vi "Dashboard Main.vi"() -> ()   [LabVIEW 2013]
uses:
  <vilib>/event_ctls.llb/eventvkey.ctl
  <vilib>/Rock Robotics/WPI/Dashboard/WPI_DashboardLogging Global.vi
  <vilib>/Utility/config.llb/Write Key (String).vi
  <vilib>/Utility/config.llb/Write Key (I32).vi
  <vilib>/Utility/config.llb/NI_LVConfig.lvlib
panel:
  out "JS2 Z 2":dbl(slide) scale=-1.0..1.0 scale format="%#_2e"
  out "Joystick 4":cluster{"X":dbl, "Y":dbl}[](graph)
  out "JS1 Z 2":dbl(slide) scale=-1.0..1.0 scale format="%#_2e"
  out "Joystick 3":cluster{"X":dbl, "Y":dbl}[](graph)
  out "code":string
  out "Image Message":string="Timeout in Camera Communications"
  in  "Rec Mode":enum32{"Stop", "Record", "Playback"}(radio)
  in  "Dashboard Tab":T1(tab)
  in  "Camera Settings":T2={"Frame Rate"=30, "Compression"=30, "Size"=1} {"Frame Rate" scale=1.0..30.0; "Size" items=["640x480", "320x240", "160x120"]}
  out "MotorSliders R":cluster{"MotorSlide1":dbl, "MotorSlide2":dbl} {"MotorSlide2" scale=-1.0..1.0 scale format="%#_2e"; "MotorSlide1" scale=-1.0..1.0 scale format="%#_2e"}
  out "MotorChart R":cluster{"Numeric":dbl, "Numeric":dbl}(graph)
  out "MotorSliders L":T3 {"MotorSlide4 2" scale=0.0..14.0 scale format="%#_2e"; "MotorSlide2" scale=-1.0..1.0 scale format="%#_2e"; "MotorSlide1" scale=-1.0..1.0 scale format="%#_2e"}
  out "MotorChart L":T4(graph)
  out "JS1 Z":dbl(slide) scale=-1.0..1.0 scale format="%#_2e"
  out "Joystick 1":cluster{"X":dbl, "Y":dbl}[](graph)
  out "JS Buttons 1":T5
  out "JS2 Z":dbl(slide) scale=-1.0..1.0 scale format="%#_2e"
  out "Joystick 2":cluster{"X":dbl, "Y":dbl}[](graph)
  out "JS Buttons 2":T5
  out "Mode":T6(ring)=enum."Auto Disabled"
  out "Camera IP":string
  in  "DB Camera Config":bool
  out "fps":dbl format="%#.1g"
  out "Mbps":dbl format="%#.1g"
  out "Mbps 2":bool
  out "LED 1":bool
  in  "loadCode":bool
  in  "pick auto":string
  out "Timer":dbl
  out "Mode 2":string
  out "left Encoder":dbl
  out "right Encoder":dbl
  out "Waveform Chart":T7(graph)
  out "Plot 0 Ind":dbl
  out "Plot 1 Ind":dbl
  out "Polt 2 Ind":dbl
  in  "Checkbox 2":bool
  in  "Checkbox 1":bool
  in  "Test Slider":dbl(slide) scale=0.0..100.0 scale format="%#_3g"
  in  "On/Off":bool caption="Solenoid"
  in  "Test Name":u16(ring) items=["Select the test to run...", "Example Test", "-------------------------------", "List of tests is built in robot code.", "Replace with your own automated tests."]
  in  "Test Tree":string(tree)
  in  "Motor":cluster{"Value":dbl, "Enable":bool} {"Value" scale=-1.0..1.0 scale format="%#_3g"}
  out "Progress":T8 {"Test Progress" scale=0.0..100.0}
  in  "Rev/Fwd":cluster{"Forward":bool, "Reverse":bool}
  in  "Test Ring":u16(ring) items=["Auto", "Fixed indoor", "Fixed outdoor 1", "Fixed outdoor 2", "Fixed fluorescent 1", "Fixed fluorescent 2", "Hold current"]
  in  "Listbox":i32(listbox)
  out "Tree":string(tree)
  out "Camera Image":T9(plugin-control)
  in  "Enable":bool
  # "Left"
  # "Front"
  # "Right"
  # "Battery"
  # "This tab is a great place for autonomous settings and validation.\nCustomize by placing controls and indicators here and name to\nmatch Dashboard Variables on robot."
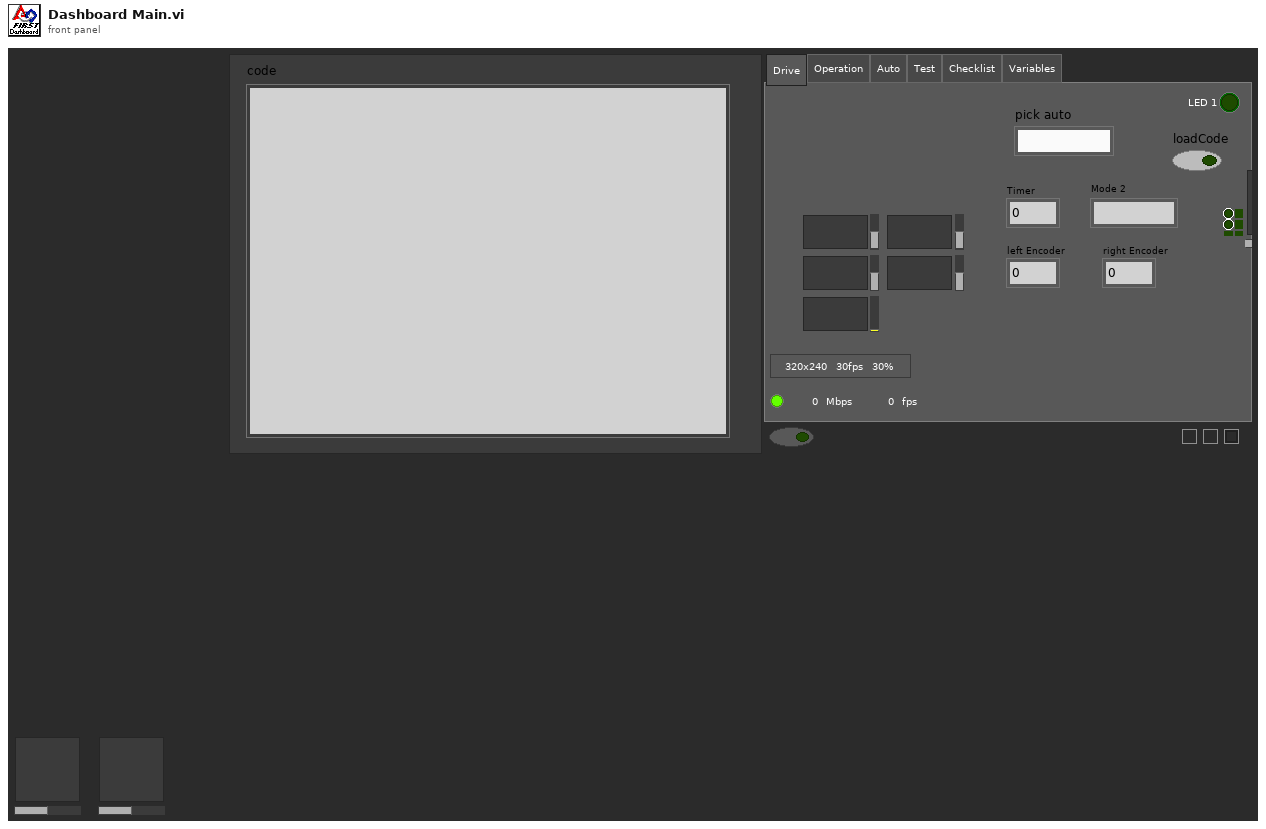
[diagram p1: front panel]
types:
  T1 = enum32{"Drive", "Operation", "Auto", "Test", "Checklist", "Variables"}
  T2 = cluster{"Frame Rate":i32, "Compression":i32, "Size":u16}
  T3 = cluster{"MotorSlide1":dbl, "MotorSlide2":dbl, "MotorSlide4 2":dbl}
  T4 = cluster{"Numeric":dbl, "Numeric":dbl, "Battery":sgl}
  T5 = cluster{bool, bool, bool, bool, bool, bool, bool, bool, bool, bool, bool, bool}
  T6 = enum8{"Tele-Op Disabled", "Tele-Op Enabled", "Auto Disabled", "Auto Enabled", "Test Disabled", "Test Enabled", ""}
  T7 = cluster{"Numeric":dbl, "Numeric":dbl, "Numeric":dbl}
  T8 = cluster{"Test Progress":u8, "Test Progress Text":string}
  T9 = typedef "IMAQ Image.ctl" = refnum<image>
  T10 = typedef "Image Type" = u32
  T11 = cluster{"Digital Inputs":bool[], "Digital Outputs":bool[]}
  T12 = cluster{"Competition mode":bool, "Robot Link":bool, "Autonomous":bool, "Enabled":bool, "E-Stop":bool, "Simulated":bool, "TestMode":bool, "Docked Window":bool}
  T13 = cluster{"Boolean":bool, "Boolean":bool, "Boolean":bool, "Boolean":bool, "Boolean":bool, "Boolean":bool, "Boolean":bool, "Boolean":bool, "Boolean":bool, "Boolean":bool, "Boolean":bool, "Boolean":bool}
  T14 = typedef "NI_LVConfig.lvlib/Config Data RefNum.ctl" = refnum<k1>
  T15 = typedef "eventvkey.ctl" = enum16{"ASCII", "Enter", "Return", "Shift", "Ctrl", "Alt", "Cmd", "Opt", "Caps", "NumLock", "Clear", "Break", "Up", "Down", "Left", "Right", "Insert", "Delete", "Home", "End", "PageUp", "PageDown", "Escape", "Help", "Pause", "ScrollLock", "F1", "F2", "F3", "F4", "F5", "F6", "F7", "F8", "F9", "F10", "F11", "F12", "F13", "F14", "F15", "F16", "F17", "F18", "F19", "F20", "F21", "F22", "F23", "F24", "Play", "VolumeUp", "VolumeDown", "Mute", "Two Byte Char"}
  T16 = cluster{"Image Size":bool, "Image Type":bool, "Pixel Value":bool, "ROI Information":bool, "Zoom Factor":bool}
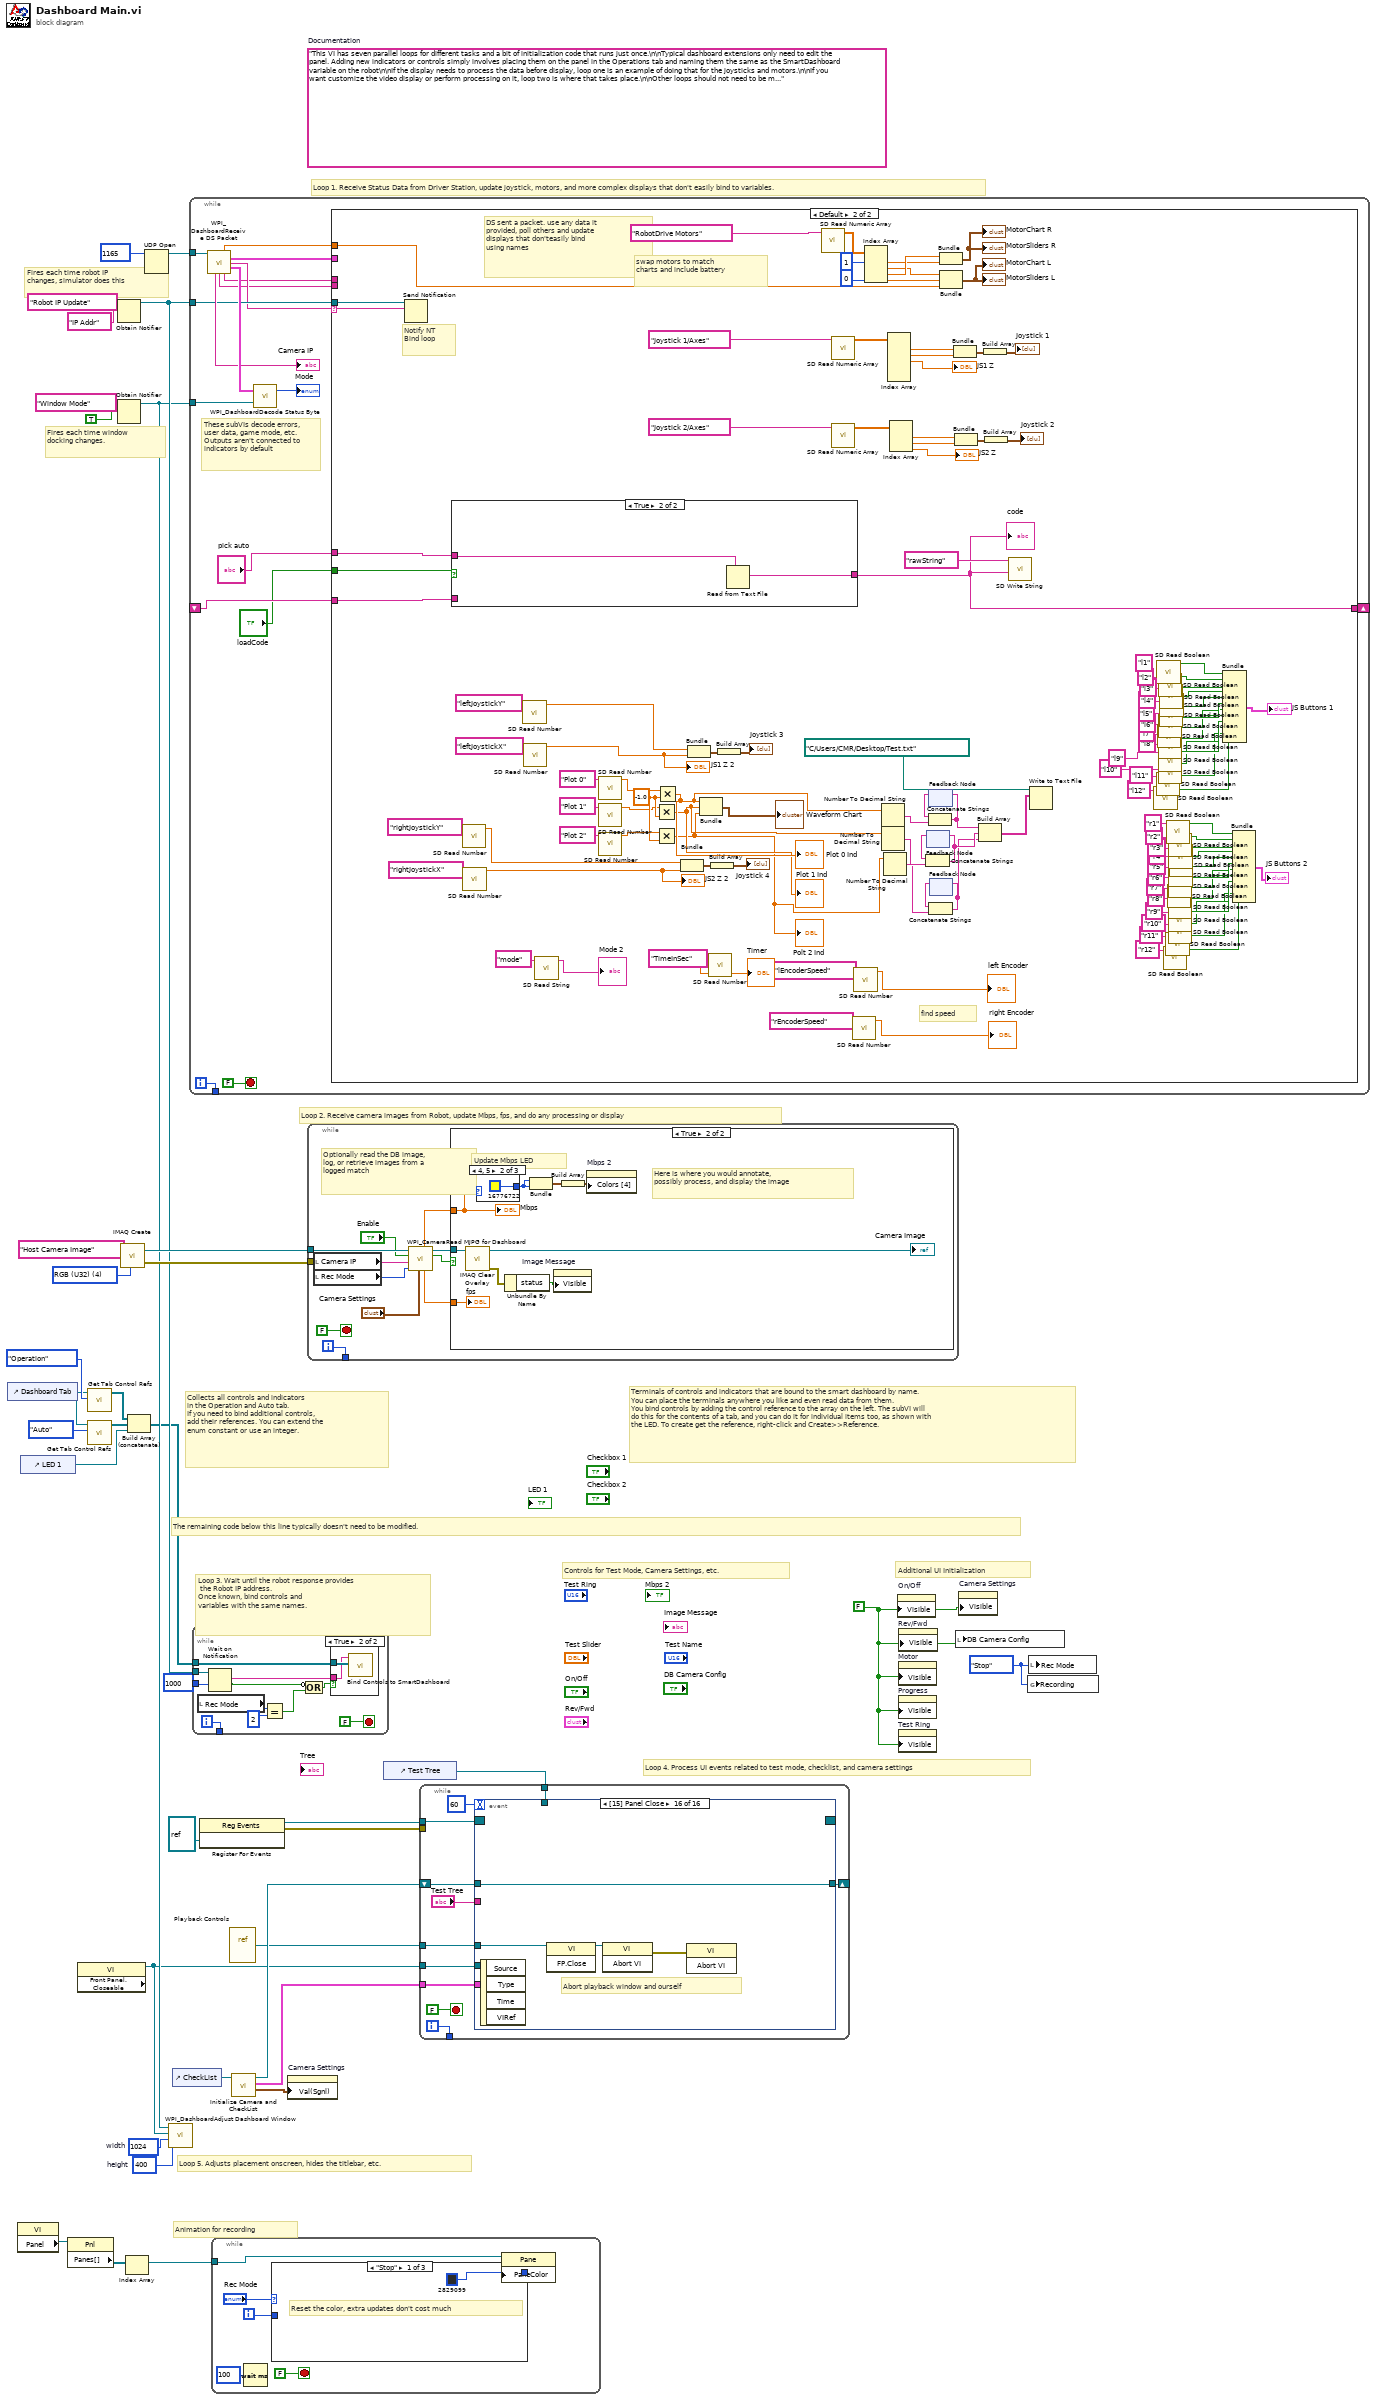
[diagram p0: block diagram]
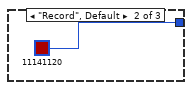
[diagram p2: hidden frame]
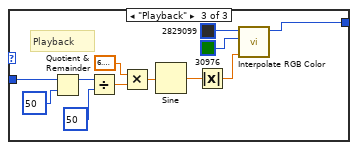
[diagram p3: hidden frame]
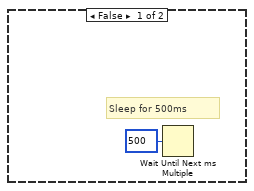
[diagram p5: hidden frame]
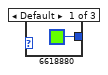
[diagram p6: hidden frame]
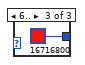
[diagram p7: hidden frame]
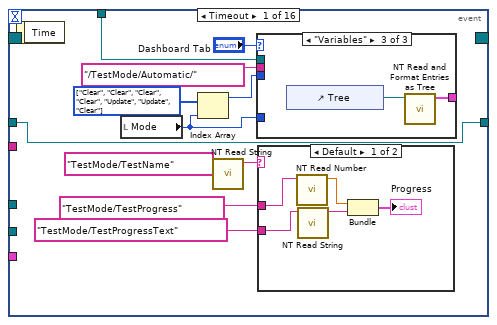
[diagram p8: hidden frame]
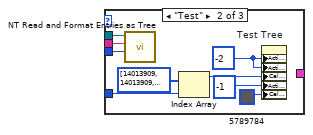
[diagram p10: hidden frame]
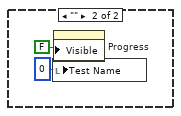
[diagram p11: hidden frame]
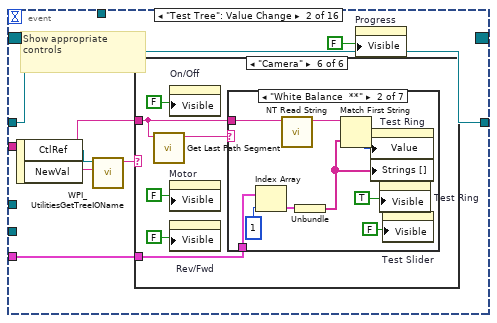
[diagram p12: hidden frame]
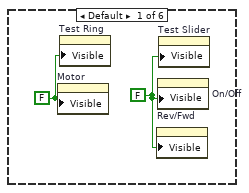
[diagram p13: hidden frame]
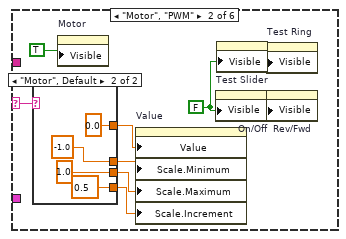
[diagram p14: hidden frame]
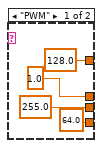
[diagram p15: hidden frame]
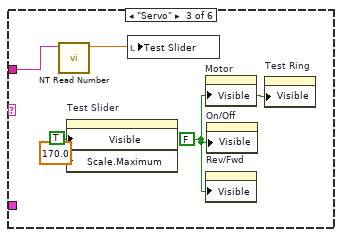
[diagram p16: hidden frame]
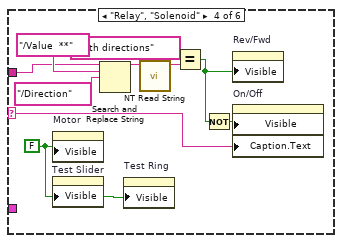
[diagram p17: hidden frame]
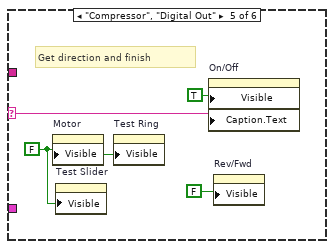
[diagram p18: hidden frame]
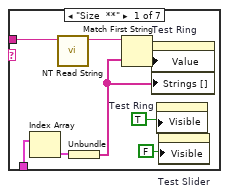
[diagram p19: hidden frame]
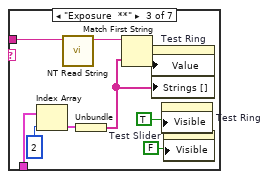
[diagram p20: hidden frame]
diagram:
  w8 = enum32{"Stop", "Record", "Playback"}."Stop" ("Rec Mode")
  w11 = 400  # height
  w12 = 1024  # width
  w25 = FALSE ("Visible")
  (unwired) "This VI has seven parallel loops for different tasks and a bit of initialization code that runs just once.\n\nTypical dashboard extensions only need to edit the panel. Adding new indicators or controls simply involves placing them on the panel in the Operations tab and naming them the same as the SmartDashboard variable on the robot\n\nIf the display needs to process the data before display, loop one is an example of doing that for the joysticks and motors.\n\nIf you want customize the video display or perform processing on it, loop two is where that takes place.\n\nOther loops should not need to be modified. They are pretty standard, and document the task they perform."  # Documentation
  w35 = T10 4 items=["Grayscale (U8)", "Grayscale (I16)", "Grayscale (SGL)", "Complex (CSG)", "RGB (U32)", "HSL (U32)", "RGB (U64)"] ("Image Type")
  # "Controls for Test Mode, Camera Settings, etc."
  # "Additional UI Initialization"
  # "Animation for recording"
  # "Fires each time robot IP\nchanges, simulator does this"
  # "Fires each time window\ndocking changes."
  # "Collects all controls and indicators\nin the Operation and Auto tab.\nIf you need to bind additional controls,\nadd their references. You can extend the\nenum constant or use an integer."
  # "The remaining code below this line typically doesn't need to be modified."
  # "Loop 4. Process UI events related to test mode, checklist, and camera settings"
  # "Terminals of controls and indicators that are bound to the smart dashboard by name.\nYou can place the terminals anywhere you like and even read data from them.\nYou bind controls by adding the control reference to the array on the left. The subVI will\ndo this for the contents of a tab, and you can do it for individual items too, as shown with\nthe LED. To create get the reference, right-click and Create>>Reference."
  # "Loop 3. Wait until the robot response provides\n the Robot IP address.\nOnce known, bind controls and\nvariables with the same names."
  # "Loop 5. Adjusts placement onscreen, hides the titlebar, etc."
  # "Loop 1. Receive Status Data from Driver Station, update joystick, motors, and more complex displays that don't easily bind to variables."
  # "Loop 2. Receive camera images from Robot, update Mbps, fps, and do any processing or display"
  n1 = control-ref of="Dashboard Tab"() -> (w6:refnum<vi>)
  n2 = property class="VI"() -> ("Panel"=w19:refnum<vi>)  [unwired: 2 in, 2 out]
  n3 = control-ref of="LED 1"() -> (w1:refnum<vi>)
  n4 = property class="Pnl"(reference=w19) -> ("Panes[]"=w20:refnum<vi>[])  [unwired: 1 in, 2 out]
  n5 = property class="VI" props=["Front Panel.Closeable"]() -> (reference out=w7:refnum<vi>)  [unwired: 2 in, 2 out]
  n6 = call <vilib>:"Get Tab Control Refs.vi"("Page Index"=T1."Operation" ("Dashboard Tab"), "TabControl in"=w6) -> ("ControlsOnPage"=w4:refnum<vi>[])  [unwired: 9 in]
  n7 = call <vilib>:"Get Tab Control Refs.vi"("Page Index"=T1."Auto" ("Dashboard Tab"), "TabControl in"=w6) -> ("ControlsOnPage"=w5:refnum<vi>[])  [unwired: 9 in]
  n8 = Obtain Notifier(name (unnamed)="Robot IP Update", notification data type="IP Addr" ("name (unnamed)")) -> (notifier out=w29:refnum<notifier>)  [unwired: 2 in, 2 out]
  n9 = Obtain Notifier(name (unnamed)="Window Mode", notification data type=TRUE) -> (notifier out=w10:refnum<notifier>)  [unwired: 2 in, 2 out]
  n10 = call "IMAQ Create"("Image Name"="Host Camera Image", "Image Type"=w35) -> ("New Image"=w33:T9, "error out"=w32:errorcluster)  [unwired: 2 in, 1 out]
  n11 = Index Array(array=w20) -> (element=w18:refnum<vi>)  [unwired: 1 in]
  n12 = Build Array (concatenate)(w4, w5, w1) -> (w3:refnum<vi>[])
  n13 = UDP Open(11:u16 1165 ("port")) -> (port=w36:refnum<k16>)  [unwired: 2 in, 4 out]
  n14 = call <vilib>:"WPI_DashboardAdjust Dashboard Window.vi"("height"=w11, "width"=w12, "reference in"=w7, "Notifier in"=w10) -> ()  [unwired: 8 in]
  n15 = control-ref of="CheckList"() -> (w9:refnum<vi>)
  n16 = while {
    tunnel: w36 -> [w53]
    tunnel: w29 -> [w48]
    tunnel: w10 -> [w52]
    tunnel: [w49] -> _
    shift-right: [w40] -> _
    shift-left: _ -> [w41]
    i -> [w49]
    stop <- FALSE stop-if-true
    # "These subVIs decode errors, user data, game mode, etc.\nOutputs aren't connected to indicators by default"
    n17 = call <vilib>:"WPI_DashboardReceive DS Packet.vi"("Recv Socket"=w53) -> ("Battery"=w43:sgl, "Driver Station"=w44:T11, "Robot IP Address"=w47:string, "Status"=w54:T12, "Camera IP Address"=→"Camera IP":string, "Low Priority User Data"=w46:string, "High Priority User Data"=w45:string)  [unwired: 1 in, 7 out]
    n18 = call <vilib>:"WPI_DashboardDecode Status Byte.vi"("Window Mode Notifier"=w52, "Status"=w54) -> ("Mode"=→"Mode":T6)  [unwired: 1 out]
    n19 = case shown="Default" w47 {
      selector: w47 -> [_ w161]
      tunnel: w48 -> [_ w162]
      tunnel: w46 -> [_ _]
      tunnel: w45 -> [_ _]
      tunnel: w44 -> [_ _]
      tunnel: w43 -> [_ w160]
      tunnel: w41 -> [w55 w149]
      tunnel: [w55 w146] -> w40
      tunnel: "pick auto" -> [_ w148]
      tunnel: "loadCode" -> [_ w147]
      frame "0.0.0.0" {
        # "DS not sending packets, or no robot exists yet.\nDon't poll the variables"
      }
      frame Default {
        w76 = -1.0 ("y")
        (unwired) "leftJoystickY" ("Name")
        (unwired) "l1" ("Name")
        # "find speed"
        # "Notify NT\nBind loop"
        # "DS sent a packet. use any data it\nprovided, poll others and update\ndisplays that don'teasily bind\nusing names"
        # "swap motors to match\ncharts and include battery"
        n20 = Send Notification(notification=w161, notifier=w162) -> ()  [unwired: 1 in, 2 out]
        n21 = case shown="True" w147 {
          tunnel: [w178 w180] -> w146
          tunnel: w149 -> [w178 _]
          tunnel: w148 -> [_ w179]
          frame False {
          }
          frame True {
            n22 = Read from Text File(prompt (Open existing file)=w179) -> (text=w180:string)  [unwired: 3 in, 3 out]
          }
        }
        "code" <- w146
        n23 = call <vilib>:"SD Read Number.vi"("Name"="rightJoystickY") -> ("Numeric"=w79:dbl)  [unwired: 8 in, 2 out]
        n24 = call <vilib>:"SD Read Number.vi"("Name"="rightJoystickX") -> ("Numeric"=w92:dbl)  [unwired: 8 in, 2 out]
        "JS2 Z 2" <- w92
        n25 = call <vilib>:"SD Read Number.vi"() -> ("Numeric"=w56:dbl)  [unwired: 9 in, 2 out]
        n26 = call <vilib>:"SD Read Number.vi"("Name"="leftJoystickX") -> ("Numeric"=w91:dbl)  [unwired: 8 in, 2 out]
        "JS1 Z 2" <- w91
        n27 = call <vilib>:"SD Read String.vi"("Name"="mode") -> ("String"=→"Mode 2":string)  [unwired: 8 in, 2 out]
        n28 = call <vilib>:"SD Read Number.vi"("Name"="Plot 0") -> ("Numeric"=w78:dbl)  [unwired: 8 in, 2 out]
        n29 = call <vilib>:"SD Read Number.vi"("Name"="Plot 1") -> ("Numeric"=w74:dbl)  [unwired: 8 in, 2 out]
        n30 = call <vilib>:"SD Read Number.vi"("Name"="Plot 2") -> ("Numeric"=w77:dbl)  [unwired: 8 in, 2 out]
        n31 = Multiply(x=w74, y=w76) -> (x*y=w71:dbl)
        "Plot 1 Ind" <- w71
        n32 = Multiply(x=w77, y=w76) -> (x*y=w70:dbl)
        "Polt 2 Ind" <- w70
        n33 = Multiply(x=w78, y=w76) -> (x*y=w72:dbl)
        "Plot 0 Ind" <- w72
        n34 = Bundle("Numeric"=w79, "Numeric"=w92) -> (w97:cluster{"Numeric":dbl, "Numeric":dbl})  [unwired: 1 in]
        n35 = Bundle("Numeric"=w56, "Numeric"=w91) -> (w99:cluster{"Numeric":dbl, "Numeric":dbl})  [unwired: 1 in]
        n36 = Bundle(w72, w71, w70) -> (→"Waveform Chart":cluster{dbl, dbl, dbl})  [unwired: 1 in]
        n37 = call <vilib>:"SD Read Number.vi"("Name"="TimeInSec") -> ("Numeric"=→"Timer":dbl)  [unwired: 8 in, 2 out]
        n38 = Build Array(w97) -> (→"Joystick 4":cluster{"Numeric":dbl, "Numeric":dbl}[])
        n39 = Build Array(w99) -> (→"Joystick 3":cluster{"Numeric":dbl, "Numeric":dbl}[])
        n40 = call <vilib>:"SD Read Numeric Array.vi"("Name"="RobotDrive Motors") -> ("Numeric Array"=w159:dbl[])  [unwired: 8 in, 2 out]
        n41 = call <vilib>:"SD Read Numeric Array.vi"("Name"="Joystick 1/Axes") -> ("Numeric Array"=w175:dbl[])  [unwired: 8 in, 2 out]
        n42 = call <vilib>:"SD Read Numeric Array.vi"("Name"="Joystick 2/Axes") -> ("Numeric Array"=w169:dbl[])  [unwired: 8 in, 2 out]
        n43 = call <vilib>:"SD Read Number.vi"("Name"="rEncoderSpeed") -> ("Numeric"=→"right Encoder":dbl)  [unwired: 8 in, 2 out]
        n44 = call <vilib>:"SD Read Number.vi"("Name"="lEncoderSpeed") -> ("Numeric"=→"left Encoder":dbl)  [unwired: 8 in, 2 out]
        n45 = Index Array(array=w159, index #1=1, index #4=0) -> (element #1=w155:dbl, element #2=w154:dbl, element #3=w156:dbl, element #4=w151:dbl)  [unwired: 2 in]
        n46 = Number To Decimal String(number=w72) -> (decimal integer string=w68:string)  [unwired: 1 in]
        n47 = Number To Decimal String(number=w71) -> (decimal integer string=w65:string)  [unwired: 1 in]
        n48 = Number To Decimal String(number=w70) -> (decimal integer string=w62:string)  [unwired: 1 in]
        n49 = Index Array(array=w175) -> (element #1=w172:dbl, element #2=w173:dbl, element #3=→"JS1 Z":dbl)  [unwired: 6 in, 3 out]
        n50 = Index Array(array=w169) -> (element #1=w166:dbl, element #2=w165:dbl, element #3=→"JS2 Z":dbl)  [unwired: 3 in]
        n51 = feedback #1() -> (w66:string)  [unwired: 1 in]
        n52 = Concatenate Strings(w66, w65) -> (w64:string)
        n53 = feedback-in #1(w64) -> ()
        n54 = feedback #2() -> (w69:string)  [unwired: 1 in]
        n55 = Concatenate Strings(w69, w68) -> (w67:string)
        n56 = feedback-in #2(w67) -> ()
        n57 = feedback #3() -> (w63:string)  [unwired: 1 in]
        n58 = Concatenate Strings(w63, w62) -> (w61:string)
        n59 = feedback-in #3(w61) -> ()
        n60 = Bundle("Numeric"=w156, "Numeric"=w155) -> (→"MotorChart R" →"MotorSliders R":cluster{"Numeric":dbl, "Numeric":dbl})  [unwired: 1 in]
        n61 = Bundle("Numeric"=w154, "Numeric"=w151, "Battery"=w160) -> (→"MotorChart L" →"MotorSliders L":T4)  [unwired: 1 in]
        n62 = Bundle("Numeric"=w172, "Numeric"=w173) -> (w171:cluster{"Numeric":dbl, "Numeric":dbl})  [unwired: 1 in]
        n63 = Bundle("Numeric"=w166, "Numeric"=w165) -> (w167:cluster{"Numeric":dbl, "Numeric":dbl})  [unwired: 1 in]
        n64 = Build Array(w67, w64, w61) -> (w60:string[])
        n65 = Build Array(w171) -> (→"Joystick 1":cluster{"Numeric":dbl, "Numeric":dbl}[])
        n66 = Build Array(w167) -> (→"Joystick 2":cluster{"Numeric":dbl, "Numeric":dbl}[])
        n67 = call <vilib>:"SD Write String.vi"("String"=w146, "Name"="rawString") -> ()  [unwired: 8 in, 2 out]
        n68 = Write to Text File(file (use dialog)=path "C:/Users/CMR/Desktop/Test.txt", text=w60) -> ()  [unwired: 2 in, 3 out]
        n69 = call <vilib>:"SD Read Boolean.vi"("Name"="l12") -> ("Boolean"=w123:bool)  [unwired: 8 in, 2 out]
        n70 = call <vilib>:"SD Read Boolean.vi"("Name"="l11") -> ("Boolean"=w124:bool)  [unwired: 8 in, 2 out]
        n71 = call <vilib>:"SD Read Boolean.vi"() -> ("Boolean"=w57:bool)  [unwired: 9 in, 2 out]
        n72 = call <vilib>:"SD Read Boolean.vi"("Name"="l7") -> ("Boolean"=w128:bool)  [unwired: 8 in, 2 out]
        n73 = call <vilib>:"SD Read Boolean.vi"("Name"="l2") -> ("Boolean"=w133:bool)  [unwired: 8 in, 2 out]
        n74 = call <vilib>:"SD Read Boolean.vi"("Name"="l6") -> ("Boolean"=w129:bool)  [unwired: 8 in, 2 out]
        n75 = call <vilib>:"SD Read Boolean.vi"("Name"="l8") -> ("Boolean"=w127:bool)  [unwired: 8 in, 2 out]
        n76 = call <vilib>:"SD Read Boolean.vi"("Name"="l9") -> ("Boolean"=w126:bool)  [unwired: 8 in, 2 out]
        n77 = call <vilib>:"SD Read Boolean.vi"("Name"="l10") -> ("Boolean"=w125:bool)  [unwired: 8 in, 2 out]
        n78 = call <vilib>:"SD Read Boolean.vi"("Name"="l3") -> ("Boolean"=w132:bool)  [unwired: 8 in, 2 out]
        n79 = call <vilib>:"SD Read Boolean.vi"("Name"="l5") -> ("Boolean"=w130:bool)  [unwired: 8 in, 2 out]
        n80 = call <vilib>:"SD Read Boolean.vi"("Name"="l4") -> ("Boolean"=w131:bool)  [unwired: 8 in, 2 out]
        n81 = call <vilib>:"SD Read Boolean.vi"("Name"="r12") -> ("Boolean"=w134:bool)  [unwired: 8 in, 2 out]
        n82 = call <vilib>:"SD Read Boolean.vi"("Name"="r11") -> ("Boolean"=w135:bool)  [unwired: 8 in, 2 out]
        n83 = call <vilib>:"SD Read Boolean.vi"("Name"="r1") -> ("Boolean"=w145:bool)  [unwired: 8 in, 2 out]
        n84 = call <vilib>:"SD Read Boolean.vi"("Name"="r7") -> ("Boolean"=w139:bool)  [unwired: 8 in, 2 out]
        n85 = call <vilib>:"SD Read Boolean.vi"("Name"="r2") -> ("Boolean"=w144:bool)  [unwired: 8 in, 2 out]
        n86 = call <vilib>:"SD Read Boolean.vi"("Name"="r6") -> ("Boolean"=w140:bool)  [unwired: 8 in, 2 out]
        n87 = call <vilib>:"SD Read Boolean.vi"("Name"="r8") -> ("Boolean"=w138:bool)  [unwired: 8 in, 2 out]
        n88 = call <vilib>:"SD Read Boolean.vi"("Name"="r9") -> ("Boolean"=w137:bool)  [unwired: 8 in, 2 out]
        n89 = call <vilib>:"SD Read Boolean.vi"("Name"="r10") -> ("Boolean"=w136:bool)  [unwired: 8 in, 2 out]
        n90 = call <vilib>:"SD Read Boolean.vi"("Name"="r3") -> ("Boolean"=w143:bool)  [unwired: 8 in, 2 out]
        n91 = call <vilib>:"SD Read Boolean.vi"("Name"="r5") -> ("Boolean"=w141:bool)  [unwired: 8 in, 2 out]
        n92 = call <vilib>:"SD Read Boolean.vi"("Name"="r4") -> ("Boolean"=w142:bool)  [unwired: 8 in, 2 out]
        n93 = Bundle("Boolean"=w57, "Boolean"=w133, "Boolean"=w132, "Boolean"=w131, "Boolean"=w130, "Boolean"=w129, "Boolean"=w128, "Boolean"=w127, "Boolean"=w126, "Boolean"=w125, "Boolean"=w124, "Boolean"=w123) -> (→"JS Buttons 1":T13)  [unwired: 1 in]
        n94 = Bundle("Boolean"=w145, "Boolean"=w144, "Boolean"=w143, "Boolean"=w142, "Boolean"=w141, "Boolean"=w140, "Boolean"=w139, "Boolean"=w138, "Boolean"=w137, "Boolean"=w136, "Boolean"=w135, "Boolean"=w134) -> (→"JS Buttons 2":T13)  [unwired: 1 in]
      }
    }
  }
  n95 = while {
    tunnel: w3 -> [w191]
    tunnel: w29 -> [w190]
    tunnel: [w188] -> _
    tunnel: u32 1000 ("milliseconds to wait") -> [w187]
    i -> [w188]
    stop <- FALSE stop-if-true
    n96 = local read "Rec Mode"() -> (w183:enum32{"Stop", "Record", "Playback"})
    n97 = Wait on Notification(notifier=w190, timeout in ms (-1)=w187) -> (notification=w189:string, timed out?=w185:bool)  [unwired: 2 in, 2 out]
    n98 = Equal?(x=w183, y=u16 2 ("Rec Mode")) -> (x = y?=w184:bool)
    n99 = Compound Arithmetic op=OR(invert w185, w184) -> (w186:bool)
    n100 = case shown="True" w186 {
      tunnel: w191 -> [_ w193]
      tunnel: w189 -> [_ w192]
      frame False {
      }
      frame True {
        n101 = call <vilib>:"Bind Controls to SmartDashboard.vi"("Bound Control Refs"=w193, "Server IP Address"=w192) -> ()  [unwired: 10 in]
      }
    }
  }
  n102 = register-events(refnum<vi> refnum) -> (reference out=w16:refnum<event-registration>, error out=w15:errorcluster)  [unwired: 2 in]
  n103 = while {
    tunnel: w18 -> [w196]
    i -> [w199]
    stop <- FALSE stop-if-true
    n104 = Wait (ms)(milliseconds to wait=u32 100) -> ()  [unwired: 1 out]
    n105 = case shown="\"Stop\"" "Rec Mode" {
      tunnel: w199 -> [_ _ w213]
      tunnel: [u32 2829099 ("Base Color") u32 11141120 ("Target Color") w202] -> w195
      frame "Stop" {
        # "Reset the color, extra updates don't cost much"
      }
      frame "Record", Default {
      }
      frame "Playback" {
        # "Playback"
        n106 = Quotient & Remainder(x=w213, y=u32 50 ("milliseconds to wait")) -> (x-y*floor(x/y)=w209:u32)  [unwired: 1 out]
        n107 = Divide(x=w209, y=u32 50 ("milliseconds to wait")) -> (x/y=w206:dbl)
        n108 = Multiply(x=6.283185307179586, y=w206) -> (x*y=w211:dbl)
        n109 = Sine(x=w211) -> (sin(x)=w210:dbl)
        n110 = Absolute Value(x=w210) -> (abs(x)=w203:dbl)
        n111 = call "Interpolate RGB Color.vi"("Proportion"=w203, "Target Color"=u32 30976, "Base Color"=u32 2829099) -> ("Result Color"=w202:u32)  [unwired: 8 in]
      }
    }
    n112 = property class="Pane"(reference=w196, "PaneColor"=w195) -> ()  [unwired: 1 in, 2 out]
  }
  n113 = vi-ref "Playback Controls.vi"() -> (w17:refnum<vi>)
  n114 = call "Initialize Camera and CheckList.vi"("ListBox in"=w9) -> ("Cluster"=w23:cluster{"value":i32, "value":i32, "index":i32}, "Array"=w24:cluster{string[]}[], "File Refnum"=w22:T14)  [unwired: 8 in]
  n115 = property on="Camera Settings" class="Clust (strict)"("Val(Sgnl)"=w23) -> ()  [unwired: 2 in, 2 out]
  n116 = while {
    tunnel: w33 -> [w223]
    tunnel: w32 -> [_]
    tunnel: [w224] -> _
    i -> [w224]
    stop <- FALSE stop-if-true
    # "Optionally read the DB image,\nlog, or retrieve images from a\nlogged match"
    n117 = local read "Camera IP"() -> (w216:string)
    n118 = local read "Rec Mode"() -> (w215:enum32{"Stop", "Record", "Playback"})
    n119 = call <vilib>:"WPI_CameraRead MJPG for Dashboard.vi"("Camera Settings"="Camera Settings", "Rec Mode"=w215, "Camera IP"=w216, "Enable"="Enable", "Refnum in"=w223) -> ("Active"=w220:bool, "Refnum out"=w222:T9, "FPS"=w219:dbl, "Bandwidth (Mbps)"=w218:dbl)  [unwired: 3 in]
    n120 = case shown="True" w220 {
      tunnel: w222 -> [_ w229]
      tunnel: w218 -> [_ w228]
      tunnel: w219 -> [_ w226]
      frame False {
        # "Sleep for 500ms"
        n121 = Wait Until Next ms Multiple(millisecond multiple=u32 500) -> ()  [unwired: 1 out]
      }
      frame True {
        # "Here is where you would annotate,\npossibly process, and display the image"
        # "Update Mbps LED"
        n122 = call "IMAQ Clear Overlay"("Image"=w229) -> ("error out"=w233:errorcluster, "Image Out"=→"Camera Image":T9)  [unwired: 2 in, 7 out]
        n123 = case shown="4, 5" w228 {
          tunnel: [u32 6618880 ("Color Box") u32 16776722 ("Color Box") u32 16716800 ("Color Box")] -> w230
          frame Default {
          }
          frame 4, 5 {
          }
          frame 6.. {
          }
        }
        n124 = Unbundle By Name(w233) -> ("status"=w234:bool)
        n125 = Bundle("Color Box"=w230, "Color Box"=w230) -> (w232:cluster{"Color Box":u32, "Color Box":u32})  [unwired: 1 out]
        n126 = property on="Image Message" class="Str"("Visible"=w234) -> ()  [unwired: 2 in, 2 out]
        n127 = Build Array(w232) -> (w231:cluster{"Color Box":u32, "Color Box":u32}[])
        n128 = property on="Mbps 2" class="Bool (strict)"("Colors [4]"=w231) -> ()  [unwired: 2 in, 2 out]
        "Mbps" <- w228
        "fps" <- w226
      }
    }
  }
  n129 = control-ref of="Test Tree"() -> (w21:refnum<vi>)
  n130 = while {
    tunnel: w24 -> [w246]
    shift-right: [w245] -> _
    shift-left: w22 -> [w244]
    tunnel: [w243] -> _
    tunnel: w21 -> [w242]
    tunnel: w17 -> [w241]
    tunnel: w16 -> [w240]
    tunnel: w15 -> [_]
    tunnel: w7 -> [w239]
    i -> [w243]
    stop <- FALSE stop-if-true
    n131 = event shown="[15] Panel Close" {
      selector: w240 -> [_ _ _ _ _ _ _ _ _ _ _ _ _ _ _ _]
      dyn-events: [_ _ _ _ _ _ _ _ _ _ _ _ _ w483 _ _] -> _
      timeout: u32 60 ("milliseconds to wait") -> [_ _ _ _ _ _ _ _ _ _ _ _ _ _ _ _]
      tunnel: w242 -> [w255 _ _ _ _ _ _ _ _ _ _ _ _ _ _ _]
      tunnel: "Test Tree" -> [_ _ _ _ _ _ _ _ w452 w460 w462 w466 w474 _ _ _]
      tunnel: w246 -> [_ w279 _ _ _ _ w416 w446 _ _ _ _ _ _ _ _]
      tunnel: [w249 w278 w377 w382 w390 w402 w415 w439 w451 w458 w461 w465 w473 w485 w499 w500] -> w245
      tunnel: w244 -> [w249 w278 w377 w382 w390 w402 w414 w439 w451 w458 w461 w465 w473 w485 w499 w500]
      tunnel: w241 -> [_ _ _ _ _ _ _ _ _ _ _ _ _ w486 _ w503]
      tunnel: w239 -> [_ _ _ _ _ _ _ _ _ _ _ _ _ w481 _ _]
      event Timeout {
        w254 = enum16{"Update", "Clear"}[] [enum."Clear", enum."Clear", enum."Clear", enum."Clear", enum."Update", enum."Update", enum."Clear"] items=["Update", "Clear"]
        n132 = event-data() -> ()  [unwired: 1 in, 1 out]
        n133 = local read "Mode"() -> (w252:T6)
        n134 = Index Array(array=w254, index=w252) -> (element=w253:enum16{"Update", "Clear"})
        n135 = call <vilib>:"NT Read String.vi"("Name"="TestMode/TestName") -> ("String"=w258:string)  [unwired: 9 in, 1 out]
        n136 = case shown="\"Variables\"" "Dashboard Tab" {
          tunnel: w255 -> [_ w268 _]
          tunnel: "/TestMode/Automatic/" ("Name Pattern") -> [_ w267 _]
          tunnel: w253 -> [_ w266 _]
          tunnel: w252 -> [_ w264 _]
          tunnel: [_ _ w270] -> _
          frame "Operation", Default {
          }
          frame "Test" {
            w263 = -2 ("Active Item:Row Number")
            n137 = call <vilib>:"NT Read and Format Entries as Tree.vi"("Operation"=w266, "Name Pattern"=w267, "Tree Refnum"=w268) -> ()  [unwired: 7 in, 2 out]
            n138 = Index Array(array=u32[] [14013909, 14013909, 14013909, 14013909, 14013909, 16777215, 14013909], index=w264) -> (element=w262:u32)
            n139 = property on="Test Tree" class="Tree (strict)"("Active Item Row Number"=w263, "ActiveColNum"=w263, "CellBG"=w262, "Active Item Row Number"=-1 ("Active Item:Row Number"), "CellBG"=u32 5789784 ("Color Box")) -> ()  [unwired: 2 in, 2 out]
          }
          frame "Variables" {
            n140 = control-ref of="Tree"() -> (w269:refnum<vi>)
            n141 = call <vilib>:"NT Read and Format Entries as Tree.vi"("Tree Refnum"=w269) -> ("Formatted Strings"=w270:cluster{"Name":string, "Value":string}[])  [unwired: 9 in, 1 out]
          }
        }
        n142 = case shown="Default" w258 {
          tunnel: "TestMode/TestProgress" ("Name") -> [w272 _]
          tunnel: "TestMode/TestProgressText" ("Name") -> [w271 _]
          frame Default {
            n143 = call <vilib>:"NT Read Number.vi"("Name"=w272) -> ("Numeric"=w273:dbl)  [unwired: 9 in, 1 out]
            n144 = call <vilib>:"NT Read String.vi"("Name"=w271) -> ("String"=w274:string)  [unwired: 9 in, 1 out]
            n145 = Bundle("Numeric"=w273, "String"=w274) -> (→"Progress":cluster{"Numeric":dbl, "String":string})  [unwired: 1 in]
          }
          frame "" {
            n146 = local write "Test Name"(u16 0) -> ()
            n147 = property on="Progress" class="Clust (strict)"("Visible"=FALSE) -> ()  [unwired: 2 in, 2 out]
          }
        }
      }
      event "Test Tree": Value Change {
        # "Show appropriate\ncontrols"
        n148 = event-data() -> ("CtlRef"=w282:refnum<vi>, "NewVal"=w280:string)  [unwired: 1 in]
        n149 = call <vilib>:"WPI_UtilitiesGetTreeIOName.vi"("NewVal"=w280, "TreeControl in"=w282) -> ("I/O Name"=w283:string)  [unwired: 9 in]
        n150 = case shown="\"Camera\"" w283 {
          selector: w283 -> [_ w290 _ w308 w317 _]
          tunnel: w280 -> [_ _ w305 w307 _ w324]
          tunnel: w279 -> [_ _ _ _ _ w323]
          frame Default {
            w285 = FALSE ("Visible")
            w284 = FALSE ("Visible")
            n151 = property on="Motor" class="Clust (strict)"("Visible"=w284) -> ()  [unwired: 2 in, 2 out]
            n152 = property on="Test Ring" class="Ring (strict)"("Visible"=w284) -> ()  [unwired: 2 in, 2 out]
            n153 = property on="Rev/Fwd" class="Clust (strict)"("Visible"=w285) -> ()  [unwired: 2 in, 2 out]
            n154 = property on="On/Off" class="Bool (strict)"("Visible"=w285) -> ()  [unwired: 2 in, 2 out]
            n155 = property on="Test Slider" class="Slide (strict)"("Visible"=w285) -> ()  [unwired: 2 in, 2 out]
          }
          frame "Motor", "PWM" {
            w291 = FALSE ("Visible")
            n156 = case shown="\"Motor\", Default" w290 {
              tunnel: [1.0 ("Value") -1.0 ("Value")] -> w289
              tunnel: [255.0 ("Value") 1.0 ("Value")] -> w288
              tunnel: [128.0 ("Value") 0.0 ("Value")] -> w287
              tunnel: [64.0 ("Value") 0.5 ("Value")] -> w286
              frame "PWM" {
              }
              frame "Motor", Default {
              }
            }
            n157 = property on="Motor" class="Clust (strict)"("Visible"=TRUE) -> ()  [unwired: 2 in, 2 out]
            n158 = property on="Value" class="Slide (strict)"("Value"=w287, "Scale.Minimum"=w289, "Scale.Maximum"=w288, "Scale.Increment"=w286) -> ()  [unwired: 2 in, 2 out]
            n159 = property on="On/Off" class="Bool (strict)"("Visible"=w291) -> ()  [unwired: 2 in, 2 out]
            n160 = property on="Test Slider" class="Slide (strict)"("Visible"=w291) -> ()  [unwired: 2 in, 2 out]
            n161 = property on="Test Ring" class="Ring (strict)"("Visible"=w291) -> ()  [unwired: 2 in, 2 out]
            n162 = property on="Rev/Fwd" class="Clust (strict)"("Visible"=w291) -> ()  [unwired: 2 in, 2 out]
          }
          frame "Servo" {
            w303 = FALSE ("Visible")
            n163 = call <vilib>:"NT Read Number.vi"("Name"=w305) -> ("Numeric"=w304:dbl)  [unwired: 9 in, 1 out]
            n164 = property on="Test Slider" class="Slide (strict)"("Visible"=TRUE, "Scale.Maximum"=170.0 ("Scale.Range:Maximum")) -> ()  [unwired: 2 in, 2 out]
            n165 = local write "Test Slider"(w304) -> ()
            n166 = property on="Motor" class="Clust (strict)"("Visible"=w303) -> ()  [unwired: 2 in, 2 out]
            n167 = property on="Rev/Fwd" class="Clust (strict)"("Visible"=w303) -> ()  [unwired: 2 in, 2 out]
            n168 = property on="On/Off" class="Bool (strict)"("Visible"=w303) -> ()  [unwired: 2 in, 2 out]
            n169 = property on="Test Ring" class="Ring (strict)"("Visible"=w303) -> ()  [unwired: 2 in, 2 out]
          }
          frame "Relay", "Solenoid" {
            w306 = FALSE ("Visible")
            n170 = property on="Motor" class="Clust (strict)"("Visible"=w306) -> ()  [unwired: 2 in, 2 out]
            n171 = property on="Test Slider" class="Slide (strict)"("Visible"=w306) -> ()  [unwired: 2 in, 2 out]
            n172 = Search and Replace String(input string=w307, search string="/Value  **", replace string="/Direction") -> (result string=w313:string)  [unwired: 5 in, 3 out]
            n173 = property on="Test Ring" class="Ring (strict)"("Visible"=w306) -> ()  [unwired: 2 in, 2 out]
            n174 = call <vilib>:"NT Read String.vi"("Name"=w313) -> ("String"=w311:string)  [unwired: 9 in, 1 out]
            n175 = Equal?(x="Both directions", y=w311) -> (x = y?=w309:bool)
            n176 = Not(x=w309) -> (.not. x?=w310:bool)
            n177 = property on="Rev/Fwd" class="Clust (strict)"("Visible"=w309) -> ()  [unwired: 2 in, 2 out]
            n178 = property on="On/Off" class="Bool (strict)"("Visible"=w310, "Caption.Text"=w308) -> ()  [unwired: 2 in, 2 out]
          }
          frame "Compressor", "Digital Out" {
            w316 = FALSE ("Visible")
            # "Get direction and finish"
            n179 = property on="Motor" class="Clust (strict)"("Visible"=w316) -> ()  [unwired: 2 in, 2 out]
            n180 = property on="Test Slider" class="Slide (strict)"("Visible"=w316) -> ()  [unwired: 2 in, 2 out]
            n181 = property on="Test Ring" class="Ring (strict)"("Visible"=w316) -> ()  [unwired: 2 in, 2 out]
            n182 = property on="On/Off" class="Bool (strict)"("Visible"=TRUE, "Caption.Text"=w317) -> ()  [unwired: 2 in, 2 out]
            n183 = property on="Rev/Fwd" class="Clust (strict)"("Visible"=FALSE) -> ()  [unwired: 2 in, 2 out]
          }
          frame "Camera" {
            n184 = call <vilib>:"Get Last Path Segment.vi"("String in"=w324) -> ("String out"=w325:string)  [unwired: 10 in]
            n185 = property on="On/Off" class="Bool (strict)"("Visible"=FALSE) -> ()  [unwired: 2 in, 2 out]
            n186 = property on="Motor" class="Clust (strict)"("Visible"=FALSE) -> ()  [unwired: 2 in, 2 out]
            n187 = property on="Rev/Fwd" class="Clust (strict)"("Visible"=FALSE) -> ()  [unwired: 2 in, 2 out]
            n188 = case shown="\"White Balance  **\"" w325 {
              tunnel: w324 -> [w331 w340 w349 w358 w367 _ w373]
              tunnel: w323 -> [w329 w337 w346 w355 w364 _ _]
              frame "Size  **" {
                n189 = Index Array(array=w329) -> (element=w328:cluster{string[]})  [unwired: 1 in]
                n190 = call <vilib>:"NT Read String.vi"("Name"=w331) -> ("String"=w330:string)  [unwired: 9 in, 1 out]
                n191 = Unbundle(w328) -> (w326:string[])
                n192 = Match First String(2:w326, 3:w330) -> (0:w327:i32)  [unwired: 1 out]
                n193 = property on="Test Ring" class="Ring (strict)"("Value"=w327, "Strings []"=w326) -> ()  [unwired: 2 in, 2 out]
                n194 = property on="Test Ring" class="Ring (strict)"("Visible"=TRUE) -> ()  [unwired: 2 in, 2 out]
                n195 = property on="Test Slider" class="Slide (strict)"("Visible"=FALSE) -> ()  [unwired: 2 in, 2 out]
              }
              frame "White Balance  **" {
                n196 = Index Array(array=w337, index=1) -> (element=w338:cluster{string[]})
                n197 = call <vilib>:"NT Read String.vi"("Name"=w340) -> ("String"=w339:string)  [unwired: 9 in, 1 out]
                n198 = Unbundle(w338) -> (w335:string[])
                n199 = Match First String(2:w335, 3:w339) -> (0:w334:i32)  [unwired: 1 out]
                n200 = property on="Test Ring" class="Ring (strict)"("Value"=w334, "Strings []"=w335) -> ()  [unwired: 2 in, 2 out]
                n201 = property on="Test Ring" class="Ring (strict)"("Visible"=TRUE) -> ()  [unwired: 2 in, 2 out]
                n202 = property on="Test Slider" class="Slide (strict)"("Visible"=FALSE) -> ()  [unwired: 2 in, 2 out]
              }
              frame "Exposure  **" {
                n203 = Index Array(array=w346, index=2) -> (element=w347:cluster{string[]})
                n204 = call <vilib>:"NT Read String.vi"("Name"=w349) -> ("String"=w348:string)  [unwired: 9 in, 1 out]
                n205 = Unbundle(w347) -> (w343:string[])
                n206 = Match First String(2:w343, 3:w348) -> (0:w344:i32)  [unwired: 1 out]
                n207 = property on="Test Ring" class="Ring (strict)"("Value"=w344, "Strings []"=w343) -> ()  [unwired: 2 in, 2 out]
                n208 = property on="Test Ring" class="Ring (strict)"("Visible"=TRUE) -> ()  [unwired: 2 in, 2 out]
                n209 = property on="Test Slider" class="Slide (strict)"("Visible"=FALSE) -> ()  [unwired: 2 in, 2 out]
              }
              frame "Exposure Priority  **" {
                n210 = Index Array(array=w355, index=3) -> (element=w356:cluster{string[]})
                n211 = call <vilib>:"NT Read String.vi"("Name"=w358) -> ("String"=w357:string)  [unwired: 9 in, 1 out]
                n212 = Unbundle(w356) -> (w352:string[])
                n213 = Match First String(2:w352, 3:w357) -> (0:w353:i32)  [unwired: 1 out]
                n214 = property on="Test Ring" class="Ring (strict)"("Value"=w353, "Strings []"=w352) -> ()  [unwired: 2 in, 2 out]
                n215 = property on="Test Ring" class="Ring (strict)"("Visible"=TRUE) -> ()  [unwired: 2 in, 2 out]
                n216 = property on="Test Slider" class="Slide (strict)"("Visible"=FALSE) -> ()  [unwired: 2 in, 2 out]
              }
              frame "Color Enable  **" {
                n217 = Index Array(array=w364, index=4) -> (element=w365:cluster{string[]})
                n218 = call <vilib>:"NT Read String.vi"("Name"=w367) -> ("String"=w366:string)  [unwired: 9 in, 1 out]
                n219 = Unbundle(w365) -> (w361:string[])
                n220 = Match First String(2:w361, 3:w366) -> (0:w362:i32)  [unwired: 1 out]
                n221 = property on="Test Ring" class="Ring (strict)"("Value"=w362, "Strings []"=w361) -> ()  [unwired: 2 in, 2 out]
                n222 = property on="Test Ring" class="Ring (strict)"("Visible"=TRUE) -> ()  [unwired: 2 in, 2 out]
                n223 = property on="Test Slider" class="Slide (strict)"("Visible"=FALSE) -> ()  [unwired: 2 in, 2 out]
              }
              frame Default {
                n224 = property on="Test Ring" class="Ring (strict)"("Visible"=FALSE) -> ()  [unwired: 2 in, 2 out]
                n225 = property on="Test Slider" class="Slide (strict)"("Visible"=FALSE) -> ()  [unwired: 2 in, 2 out]
              }
              frame "Brightness  **", "Color Level  **", "Compression  **", "FPS  **", "Sharpness  **" {
                n226 = call <vilib>:"NT Read Number.vi"("Name"=w373) -> ("Numeric"=w372:dbl)  [unwired: 9 in, 1 out]
                n227 = local write "Test Slider"(w372) -> ()
                n228 = property on="Test Slider" class="Slide (strict)"("Visible"=TRUE, "Scale.Maximum"=100.0 ("Scale.Range:Maximum")) -> ()  [unwired: 2 in, 2 out]
                n229 = property on="Test Ring" class="Ring (strict)"("Visible"=FALSE) -> ()  [unwired: 2 in, 2 out]
              }
            }
          }
        }
        n230 = property on="Progress" class="Clust (strict)"("Visible"=FALSE) -> ()  [unwired: 2 in, 2 out]
      }
      event "Test Name": Mouse Enter {
        # "Populate the ring with the list of tests"
        n231 = event-data() -> ()  [unwired: 1 in, 1 out]
        n232 = call <vilib>:"NT Read String Array.vi"("Name"="TestMode/TestList") -> ("String Array"=w381:string[])  [unwired: 9 in, 1 out]
        n233 = Build Array (concatenate)("Select the test to run...", w381) -> (w380:string[])
        n234 = property on="Test Name" class="Ring (strict)"("Strings []"=w380) -> ()  [unwired: 2 in, 2 out]
      }
      event "Test Name": Value Change {
        w383 = FALSE ("Visible")
        # "Tell the robot the test name to run"
        n235 = event-data() -> ("NewVal"=w387:u16)  [unwired: 1 in]
        n236 = property on="Test Name" class="Ring (strict)"() -> ("Strings []"=w388:string[])  [unwired: 2 in, 2 out]
        n237 = local write "Progress"(T8 {"Test Progress"=0, "Test Progress Text"=""} ("Progress")) -> ()
        n238 = Index Array(array=w388, index=w387) -> (element=w386:string)
        n239 = call <vilib>:"NT Write String.vi"("String"=w386, "Name"="TestMode/TestName") -> ()  [unwired: 9 in, 1 out]
        n240 = property on="Progress" class="Clust (strict)"("Visible"=TRUE) -> ()  [unwired: 2 in, 2 out]
        n241 = property on="Motor" class="Clust (strict)"("Visible"=w383) -> ()  [unwired: 2 in, 2 out]
        n242 = property on="Test Slider" class="Slide (strict)"("Visible"=w383) -> ()  [unwired: 2 in, 2 out]
        n243 = property on="On/Off" class="Bool (strict)"("Visible"=w383) -> ()  [unwired: 2 in, 2 out]
        n244 = property on="Rev/Fwd" class="Clust (strict)"("Visible"=w383) -> ()  [unwired: 2 in, 2 out]
        n245 = property on="Test Ring" class="Ring (strict)"("Visible"=w383) -> ()  [unwired: 2 in, 2 out]
      }
      event "Listbox": Double Click {
        n246 = event-data() -> ("PlatMods.Shift"=w391:bool, "Row"=w393:i32)  [unwired: 1 in]
        n247 = case shown="True" w391 {
          tunnel: w393 -> [w397 _]
          tunnel: 1 -> [w396 _]
          frame False {
            n248 = property on="Listbox" class="LstBox (strict)"() -> ("Item Symbols"=w395:i32[])  [unwired: 2 in, 2 out]
            n249 = Replace Array Subset(array=w395, new element=w396, index=w397) -> (w394:i32[])
            n250 = property on="Listbox" class="LstBox (strict)"("Item Symbols"=w394) -> ()  [unwired: 2 in, 2 out]
          }
          frame True {
            w398 = 0 ("Top Row")
            n251 = property on="Listbox" class="LstBox (strict)"() -> ("Number of Rows"=w400:u32)  [unwired: 2 in, 2 out]
            n252 = Initialize Array(0, w400) -> (w399:i32[])
            n253 = property on="Listbox" class="LstBox (strict)"("Top Row"=w398, "Value"=w398, "Item Symbols"=w399) -> ()  [unwired: 2 in, 2 out]
          }
        }
      }
      event "Listbox": Key Down {
        n254 = event-data() -> ("VKey"=w404:T15)  [unwired: 1 in]
        n255 = case shown="\"Left\", \"Right\"" w404 {
          selector: w404 -> [w409 _]
          tunnel: eventvkey."Left" ("VKey") -> [w407 _]
          frame "Left", "Right" {
            n256 = Equal?(x=w407, y=w409) -> (x = y?=w408:bool)
            n257 = Select(t=0, s=w408, f=1) -> (s? t:f=w410:i32)
            n258 = property on="Listbox" class="LstBox (strict)"() -> ("Item Symbols"=w413:i32[])  [unwired: 2 in, 2 out]
            n259 = Replace Array Subset(array=w413, new element=w410, index="Listbox") -> (w412:i32[])
            n260 = property on="Listbox" class="LstBox (strict)"("Item Symbols"=w412) -> ()  [unwired: 2 in, 2 out]
          }
          frame Default {
          }
        }
      }
      event "DB Camera Config": Value Change {
        n261 = event-data() -> ("NewVal"=w417:bool)  [unwired: 1 in]
        n262 = case shown="False" w417 {
          tunnel: w416 -> [w426 _]
          tunnel: [w419 w437] -> w415
          tunnel: w414 -> [w418 w437]
          frame False {
            w433 = "Camera"
            w436 = FALSE ("Visible")
            n263 = local read "Camera Settings"() -> (w425:T2)
            n264 = Index Array(array=w426) -> (element=w429:cluster{string[]})  [unwired: 1 in]
            n265 = Unbundle(w425) -> ("Frame Rate"=w424:i32, "Compression"=w423:i32, "Size"=w427:u16)
            n266 = Unbundle(w429) -> (w428:string[])
            n267 = Index Array(array=w428, index=w427) -> (element=w422:string)
            n268 = call-poly <vilib>:"Write Key.vi"("section"=w433, "value"=w422, "key"="Size", "refnum"=w418) -> ("refnum out"=w435:T14)  [unwired: 2 in, 5 out]
            n269 = call-poly <vilib>:"Write Key.vi"("section"=w433, "value"=w424, "key"="FrameRate", "refnum"=w435) -> ("refnum out"=w434:T14)  [unwired: 1 in, 6 out]
            n270 = local write "DB Camera Config"(w436) -> ()
            n271 = property on="Camera Settings" class="Clust (strict)"("Visible"=w436) -> ()  [unwired: 2 in, 2 out]
            n272 = call-poly <vilib>:"Write Key.vi"("section"=w433, "value"=w423, "key"="Compression", "refnum"=w434) -> ("refnum out"=w420:T14)  [unwired: 1 in, 6 out]
            n273 = call <vilib>:"Close Config Data.vi"("refnum"=w420) -> ("file path"=w421:path)  [unwired: 2 in, 8 out]
            n274 = call <vilib>:"Open Config Data.vi"("configuration file path"=w421) -> ("refnum"=w419:T14)  [unwired: 8 in, 2 out]
          }
          frame True {
            n275 = property on="Camera Settings" class="Clust (strict)"("Visible"=TRUE) -> ()  [unwired: 2 in, 2 out]
          }
        }
      }
      event "Camera Settings": Value Change {
        n276 = event-data() -> ("NewVal"=w450:T2)  [unwired: 1 in]
        n277 = Index Array(array=w446) -> (element=w445:cluster{string[]})  [unwired: 1 in]
        n278 = Unbundle(w450) -> ("Frame Rate"=w441:i32, "Compression"=w440:i32, "Size"=w443:u16)
        n279 = Unbundle(w445) -> (w444:string[])
        n280 = Index Array(array=w444, index=w443) -> (element=w442:string)
        n281 = Format Into String(format string="%s   %dfps   %d%%", w442, w441, w440) -> (resulting string=w447:string)  [unwired: 2 in, 1 out]
        n282 = Build Array(w447) -> (w448:string[])
        n283 = property on="DB Camera Config" class="Bool (strict)"("Strings [4]"=w448) -> ()  [unwired: 2 in, 2 out]
      }
      event "Motor.Enable": Value Change {
        n284 = event-data() -> ("NewVal"=w456:bool)  [unwired: 1 in]
        n285 = Unbundle("Motor") -> ("Value"=w455:dbl)  [unwired: 1 out]
        n286 = Select(t=w455, s=w456, f=0.0) -> (s? t:f=w453:dbl)
        n287 = call <vilib>:"NT Write Number.vi"("Numeric"=w453, "Name"=w452) -> ()  [unwired: 9 in, 1 out]
      }
      event "Test Slider": Value Change {
        n288 = event-data() -> ("NewVal"=w459:dbl)  [unwired: 1 in]
        n289 = call <vilib>:"NT Write Number.vi"("Numeric"=w459, "Name"=w460) -> ()  [unwired: 9 in, 1 out]
      }
      event "On/Off": Value Change {
        n290 = event-data() -> ("NewVal"=w464:bool)  [unwired: 1 in]
        n291 = Boolean To (0,1)(Boolean=w464) -> (0, 1=w463:i16)
        n292 = call <vilib>:"NT Write Number.vi"("Numeric"=w463, "Name"=w462) -> ()  [unwired: 9 in, 1 out]
      }
      event "Rev/Fwd": Value Change {
        n293 = event-data() -> ("NewVal.Forward"=w472:bool, "NewVal.Reverse"=w471:bool)  [unwired: 1 in]
        n294 = Boolean To (0,1)(Boolean=w472) -> (0, 1=w468:i16)
        n295 = Boolean To (0,1)(Boolean=w471) -> (0, 1=w470:i16)
        n296 = Negate(x=w470) -> (-x=w469:i16)
        n297 = Add(x=w468, y=w469) -> (x+y=w467:i16)
        n298 = call <vilib>:"NT Write Number.vi"("Numeric"=w467, "Name"=w466) -> ()  [unwired: 9 in, 1 out]
      }
      event "Test Ring": Value Change {
        n299 = event-data() -> ("NewVal"=w476:u16)  [unwired: 1 in]
        n300 = property on="Test Ring" class="Ring (strict)"() -> ("Strings []"=w477:string[])  [unwired: 2 in, 2 out]
        n301 = Index Array(array=w477, index=w476) -> (element=w475:string)
        n302 = call <vilib>:"NT Write String.vi"("String"=w475, "Name"=w474) -> ()  [unwired: 9 in, 1 out]
      }
      event "Rec Mode": Value Change {
        # "Update globals for recording mode and path to read log from.\nClear when logging and let NetworkTables set path for vision to\nuse."
        n303 = event-data() -> ("NewVal"=w487:enum32{"Stop", "Record", "Playback"})  [unwired: 1 in]
        n304 = global write "WPI_DashboardLogging Global.vi" "Logging Filename"(path "") -> ()
        n305 = global write "WPI_DashboardLogging Global.vi" "Recording"(w487) -> ()
        n306 = case shown="\"Stop\", \"Record\"" w487 {
          tunnel: w486 -> [_ w489 w497]
          tunnel: [_ _ w496] -> w483
          tunnel: [_ _ w495] -> _
          tunnel: w481 -> [_ _ w493]
          tunnel: cluster{i32, i32} {-250, 170} -> [_ _ w492]
          tunnel: [_ _ T16 {"Image Size"=TRUE, "Image Type"=TRUE, "Pixel Value"=TRUE, "ROI Information"=TRUE, "Zoom Factor"=FALSE} ("Image Information Shown:All Elements")] -> w479
          tunnel: [_ _ TRUE ("Zoom Factor")] -> w478
          frame Default {
          }
          frame "Stop", "Record" {
            # "Place Window too"
            n307 = invoke class="VI" method="FP.Close"(reference=w489) -> (reference out=w488:refnum<vi>)  [unwired: 2 in, 2 out]
            n308 = invoke class="VI" method="Abort VI"(reference=w488) -> ()  [unwired: 2 in, 3 out]
          }
          frame "Playback" {
            n309 = call "Open Playback Panel.vi"("Offset"=w492, "DB VI Ref"=w493, "Playback in"=w497) -> ("Playback out"=w494:refnum<vi>)  [unwired: 8 in]
            n310 = register-events(w494) -> (reference out=w496:refnum<event-registration>, error out=w495:errorcluster)  [unwired: 2 in]
          }
        }
        n311 = property on="Camera Image" class="ImageControl"("Image Information Shown"=w479, "Image Information Visible"=w478) -> ()  [unwired: 2 in, 2 out]
        n312 = call <vilib>:"WPI_DashboardNT Log FieldName Cache.vi"("Operation"=enum16{"Lookup/Add", "Index", "Clear"}."Clear") -> ()  [unwired: 8 in, 3 out]
      }
      event Panel Close {
        w498 = enum32{"Stop", "Record", "Playback"}."Stop" ("Rec Mode")
        n313 = event-data() -> ()  [unwired: 1 in, 4 out]
        n314 = local write "Rec Mode"(w498) -> ()
        n315 = global write "WPI_DashboardLogging Global.vi" "Recording"(w498) -> ()
      }
      event Panel Close {
        # "Abort playback window and ourself"
        n316 = event-data() -> ()  [unwired: 1 in, 4 out]
        n317 = invoke class="VI" method="FP.Close"(reference=w503) -> (reference out=w502:refnum<vi>)  [unwired: 2 in, 2 out]
        n318 = invoke class="VI" method="Abort VI"(reference=w502) -> (error out=w501:errorcluster)  [unwired: 2 in, 2 out]
        n319 = invoke class="VI" method="Abort VI"(error in=w501) -> ()  [unwired: 2 in, 3 out]
      }
    }
  }
  n320 = property on="On/Off" class="Bool (strict)"("Visible"=w25) -> ()  [unwired: 2 in, 2 out]
  n321 = property on="Motor" class="Clust (strict)"("Visible"=w25) -> ()  [unwired: 2 in, 2 out]
  n322 = property on="Progress" class="Clust (strict)"("Visible"=w25) -> ()  [unwired: 2 in, 2 out]
  n323 = property on="Test Ring" class="Ring (strict)"("Visible"=w25) -> ()  [unwired: 2 in, 2 out]
  n324 = property on="Rev/Fwd" class="Clust (strict)"("Visible"=w25) -> ()  [unwired: 2 in, 2 out]
  n325 = local write "DB Camera Config"(w25) -> ()
  n326 = property on="Camera Settings" class="Clust (strict)"("Visible"=w25) -> ()  [unwired: 2 in, 2 out]
  n327 = global write "WPI_DashboardLogging Global.vi" "Recording"(w8) -> ()
  n328 = local write "Rec Mode"(w8) -> ()
